vi "lsstCommand.vi"(3 "error in (no error)":errorcluster, 7 "data":u32[](array[numeric]) format="%x", 8 "nbitems":u8, 9 "messagetype":u32, 11 "execute":bool) -> (0 "error out":errorcluster)   [LabVIEW 2014]
uses:
  GlobComm.vi
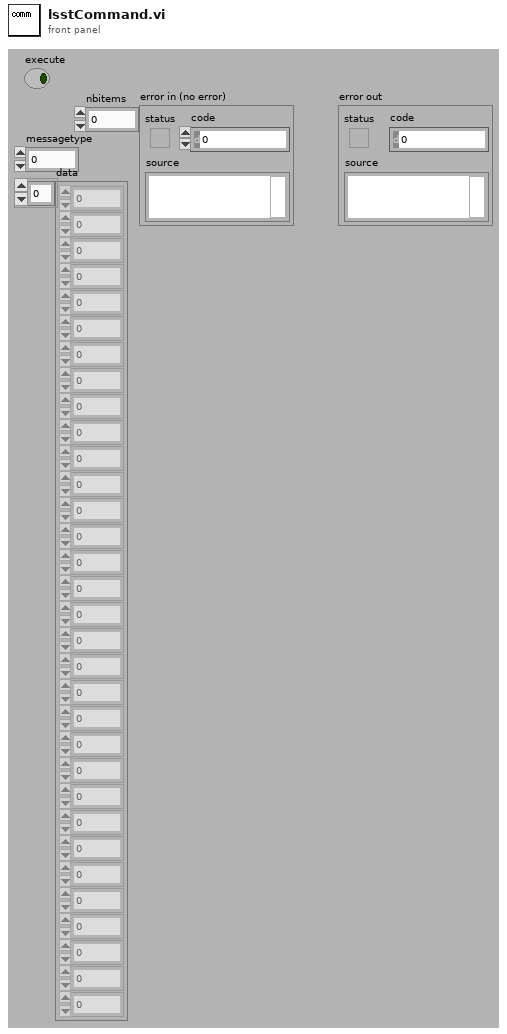
[diagram p1: front panel]
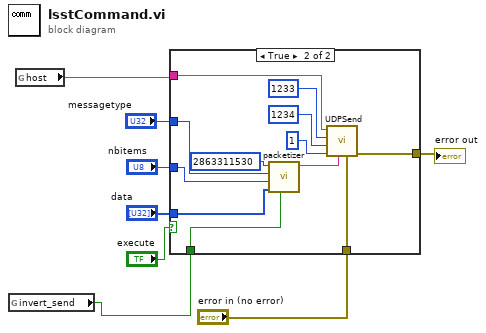
[diagram p0: block diagram]
diagram:
  n1 = global read "GlobComm.vi" "invert_send"() -> (w1:bool)
  n2 = global read "GlobComm.vi" "host"() -> (w2:string)
  n3 = case shown="True" "execute" {
    tunnel: w2 -> [_ w16]
    tunnel: "messagetype" -> [_ w15]
    tunnel: "data" -> [_ w14]
    tunnel: "nbitems" -> [_ w13]
    tunnel: "error in (no error)" -> [w9 w12]
    tunnel: [w9 w11] -> w3
    tunnel: w1 -> [_ w10]
    frame False {
    }
    frame True {
      n4 = call "packetizer.vi"("invert"=w10, "data"=w14, "countfields"=w13, "messagetype"=w15, "header"=u32 2863311530) -> ("output"=w17:string)  [unwired: 4 out]
      n5 = call "UDPSend.vi"("error in (no error)"=w12, "Data String"=w17, "# Repetitions"=1, "Remote Port"=u16 1234, "Local Port"=u16 1233, "Remote Host"=w16) -> ("error out"=w11:errorcluster)  [unwired: 2 in, 3 out]
    }
  }
  "error out" <- w3
